vi "fill_calibration_options.vi"(11 "ComboBox in":refnum<vi>) -> ()   [LabVIEW 2023]
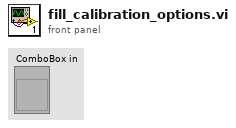
[diagram p1: front panel]
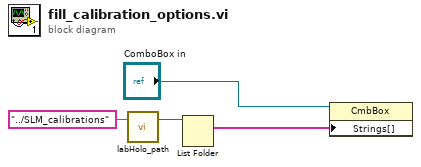
[diagram p0: block diagram]
diagram:
  n1 = call "labHolo_path.vi"("sub folder or file (str)"="../SLM_calibrations") -> ("labHolo path"=w3:path)  [unwired: 1 in, 1 out]
  n2 = List Folder(path=w3) -> (filenames=w1:string[])  [unwired: 3 in, 3 out]
  n3 = property on="Property Node" class="CmbBox"(reference="ComboBox in", "Strings[]"=w1) -> ()  [unwired: 1 in, 2 out]
